vi "Get Tagged Union Info.vi"(7 "application reference (local)":refnum<vi>, 8 "error in (no error)":errorcluster, 11 "Type in":variant) -> (0 "error out":errorcluster, 2 "Enum Type":variant, 3 "Element Types":variant[](array[variant]))   [LabVIEW 2015, in "Scripting.lvlib"]
uses:
  Scripting.lvlib
  <vilib>/Utility/Data Type/NI_Data Type.lvlib
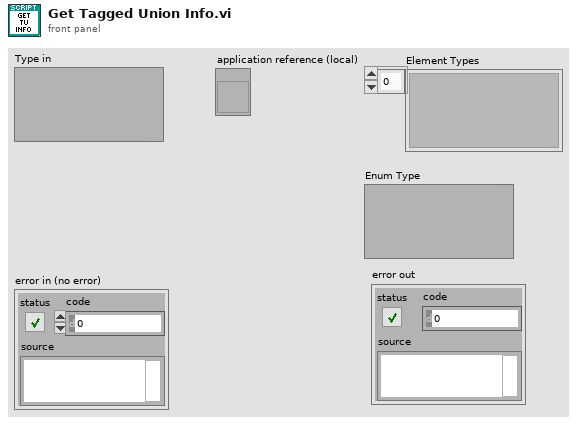
[diagram p1: front panel]
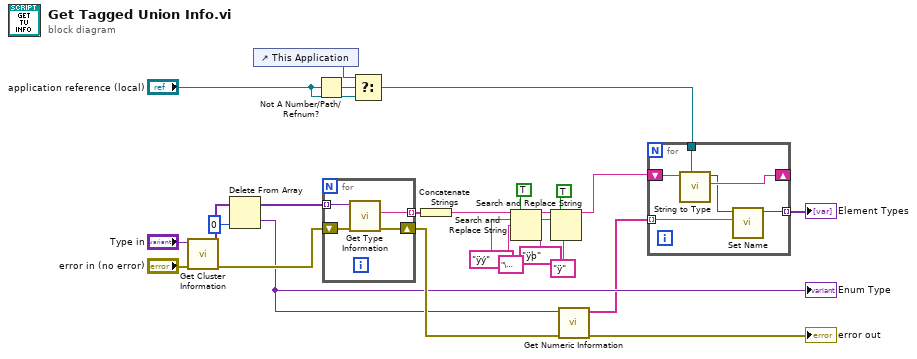
[diagram p0: block diagram]
diagram:
  n1 = call <vilib>:"Get Cluster Information.vi"("error in (no error)"="error in (no error)", "Variant"="Type in") -> ("error out"=w25:errorcluster, "Cluster Elements"=w21:variant[])  [unwired: 8 in]
  n2 = Delete From Array(array=w21, index=0) -> (deleted portion=w17:variant, array with subset deleted=w22:variant[])  [unwired: 1 in]
  "Enum Type" <- w17
  n3 = control-ref of="This Application"() -> (w3:refnum<vi>)
  n4 = Not A Number/Path/Refnum?(number/path/refnum="application reference (local)") -> (NaN/Path/Refnum?=w4:bool)
  n5 = for {
    tunnel: w22 -> [w28] mode=indexing
    tunnel: [w26] -> w18 mode=indexing
    shift-right: [w27] -> w23
    shift-left: w25 -> [w29]
    n6 = call <vilib>:"Get Type Information.vi"("error in (no error)"=w29, "Variant"=w28) -> ("error out"=w27:errorcluster, "Name"=w26:string)  [unwired: 5 in, 3 out]
  }
  n7 = Select(t=w3, s=w4, f="application reference (local)") -> (s? t:f=w1:refnum<vi>)
  n8 = Concatenate Strings(w18) -> (w7:string)
  n9 = Search and Replace String(replace all?=TRUE ("replace all? (F)"), input string=w7, search string="ÿý", replace string="\u0000" ("search string")) -> (result string=w12:string)  [unwired: 4 in, 3 out]
  n10 = Search and Replace String(replace all?=TRUE ("replace all? (F)"), input string=w12, search string="ÿþ", replace string="ÿ" ("search string")) -> (result string=w6:string)  [unwired: 4 in, 3 out]
  n11 = call <vilib>:"Get Numeric Information.vi"("error in (no error)"=w23, "Variant"=w17) -> ("error out"=→"error out":errorcluster, "Enum Names"=w16:string[])  [unwired: 6 in, 2 out]
  n12 = for {
    tunnel: w16 -> [w34] mode=indexing
    tunnel: [w33] -> w15 mode=indexing
    shift-right: [w32] -> _
    shift-left: w6 -> [w35]
    tunnel: w1 -> [w30]
    n13 = call "String to Type.vi"("application reference (local)"=w30, "String"=w35) -> ("Rest of the String"=w32:string, "Type"=w31:variant)  [unwired: 7 in, 1 out]
    n14 = call "Set Name.vi"("Name"=w34, "Type in"=w31) -> ("Type out"=w33:variant)  [unwired: 8 in, 1 out]
  }
  "Element Types" <- w15
